vi "MotorDirectControl.vi"(0 "station index":u8, 1 "Hall Positions":i32[](array[numeric]), 3 "JKI_Prefix":string="CMD-", 4 "Exit Refnum":refnum<vi>, 5 "Motion":T3, 6 "PatrType":string, 7 "AnalogData in":dbl[][](array[numeric]), 8 "Manual operation":bool, 9 "open Switch":T1={"Tag Name"="S060.PXI.Signals.PlltData.SN", "Network Path"="172.15.51.1,1,0", "use opc"=FALSE, "DataSocket Reference"={"CWDSLib._DCWDataSocket"=refnum, "CWDSLib._DCWData"=refnum, "OnDataUpdated"=0, "OnStatusUpdated"=0}} {"DataSocket Reference"."OnStatusUpdated" format="%.0x"; "DataSocket Reference"."OnDataUpdated" format="%.0x"}, 10 "test mode":bool, 11 "close Switch":T1={"Tag Name"="S060.PXI.Signals.PlltData.SN", "Network Path"="172.15.51.1,1,0", "use opc"=FALSE, "DataSocket Reference"={"CWDSLib._DCWDataSocket"=refnum, "CWDSLib._DCWData"=refnum, "OnDataUpdated"=0, "OnStatusUpdated"=0}} {"DataSocket Reference"."OnStatusUpdated" format="%.0x"; "DataSocket Reference"."OnDataUpdated" format="%.0x"}, 12 "Position Refnum":refnum<vi>) -> (13 "AnalogData out":dbl[][](array[numeric]), 14 "结果":bool, 15 "Error":string, 18 "motion str":string)   [LabVIEW 2018]
uses:
  02.Type Def's/All Motions.ctl
  05.UserVI's/type defs/plc path and tag.ctl
  <vilib>/Platform/dataskt.llb/DataSocket Reference Type.ctl
  <vilib>/Utility/error.llb/DialogType.ctl
  type def/Direct Value Mode.ctl
panel:
  out "字符串":string
  in  "Display":bool
  in  "参数设定":bool
  out "霍尔位置":i32
  out "波形图表":cluster{"玻璃当前Hall":i64, "玻璃当前Hall":sgl}(graph)
  in  "玻璃一键打开":bool
  in  "玻璃一键关闭":bool
  in  "玻璃点动打开":bool
  in  "玻璃点动关闭":bool
  in  "玻璃初始化":bool
  in  "OK":bool
  in  "打开到位置":bool
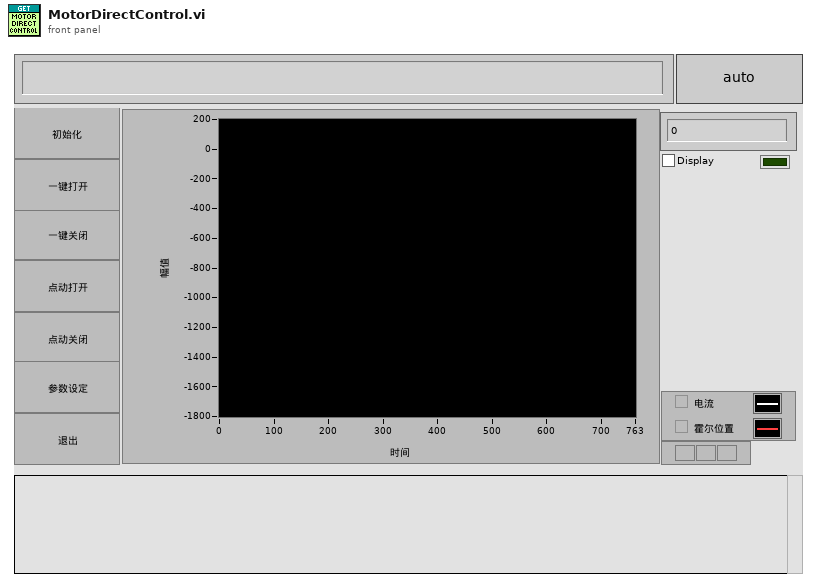
[diagram p1: front panel]
types:
  T1 = typedef "plc path and tag.ctl" = cluster{"Tag Name":string, "Network Path":string, "use opc":bool, "DataSocket Reference":T2}
  T2 = typedef "DataSocket Reference Type.ctl" = cluster{"CWDSLib._DCWDataSocket":refnum<k7>, "CWDSLib._DCWData":refnum<k7>, "OnDataUpdated":u32, "OnStatusUpdated":u32}
  T3 = typedef "All Motions.ctl" = enum16{"Glass Teach", "Glass Slide Open", "Glass Slide Close", "Glass Vent Open", "Glass Vent Close", "Sunshade Teach", "Sunshade Open", "Sunshade Close", "Idle", "Sunshade Open 2", "Sunshade Close 2", "Glass Slide Open Sunshade Open", "Glass Slide Open Sunshade Close", "Glass Slide Close Sunshade Open", "Glass Slide Close Sunshade Close", "Glass Vent Open Sunshade Open", "Glass Vent Open Sunshade Close", "Glass Vent Close Sunshade Open", "Glass Vent Close Sunshade Close", "Express Glass Slide Open", "Express Glass Slide Close", "Express Glass Vent Open", "Express Glass Vent Close", "Express Sunshade Open", "Express Sunshade Close", "Express Sunshade Open 2", "Express Sunshade Close 2", "Express Glass Slide Open Sunshade Open", "Express Glass Slide Open Sunshade Close", "Express Glass Slide Close Sunshade Open", "Express Glass Slide Close Sunshade Close", "Express Glass Vent Open Sunshade Open", "Express Glass Vent Open Sunshade Close", "Express Glass Vent Close Sunshade Open", "Express Glass Vent Close Sunshade Close", "Goto Position Glass", "Goto Position Sunshade", "Sunshade Teach 2"}
  T4 = enum32{"Invalid", "Standard", "Closed", "Hidden", "Minimized", "Maximized"}
  T5 = enum32{"invalid app kind", "Development System", "Run Time System", "Student Edition", "Embedded LabVIEW", "Evaluation", "Custom"}
  T6 = typedef "Direct Value Mode.ctl" = enum16{"Init", "read", "write send cmd", "write ER", "write position", "write AP", "write remote", "write RS", "write all input", "write Msend cmd", "write recevie cmd", "write test mode"}
  T7 = cluster{"Core":cluster{"Current VI Reference":refnum<vi>, "Close Panel on Exit?":bool}, "JKI_Prefix":string, "Hall Positions":i32[], "Action Ref":refnum<user-event>, "DerStationIndex":i32, "RunTime":i32, "Exit Refnum":refnum<vi>, "test state":bool, "current step":string, "Error":string, "Mode":bool, "Manual Operator":bool, "motion string":string, "AnalogData":dbl[][], "station index":i32, "dataNO.":i32, "Position Refnum":refnum<vi>, "Action Switch":T1, "Stop Switch":T1}
  T8 = typedef "DialogType.ctl" = u16
  T9 = cluster{"Current VI Reference":refnum<vi>, "Close Panel on Exit?":bool}
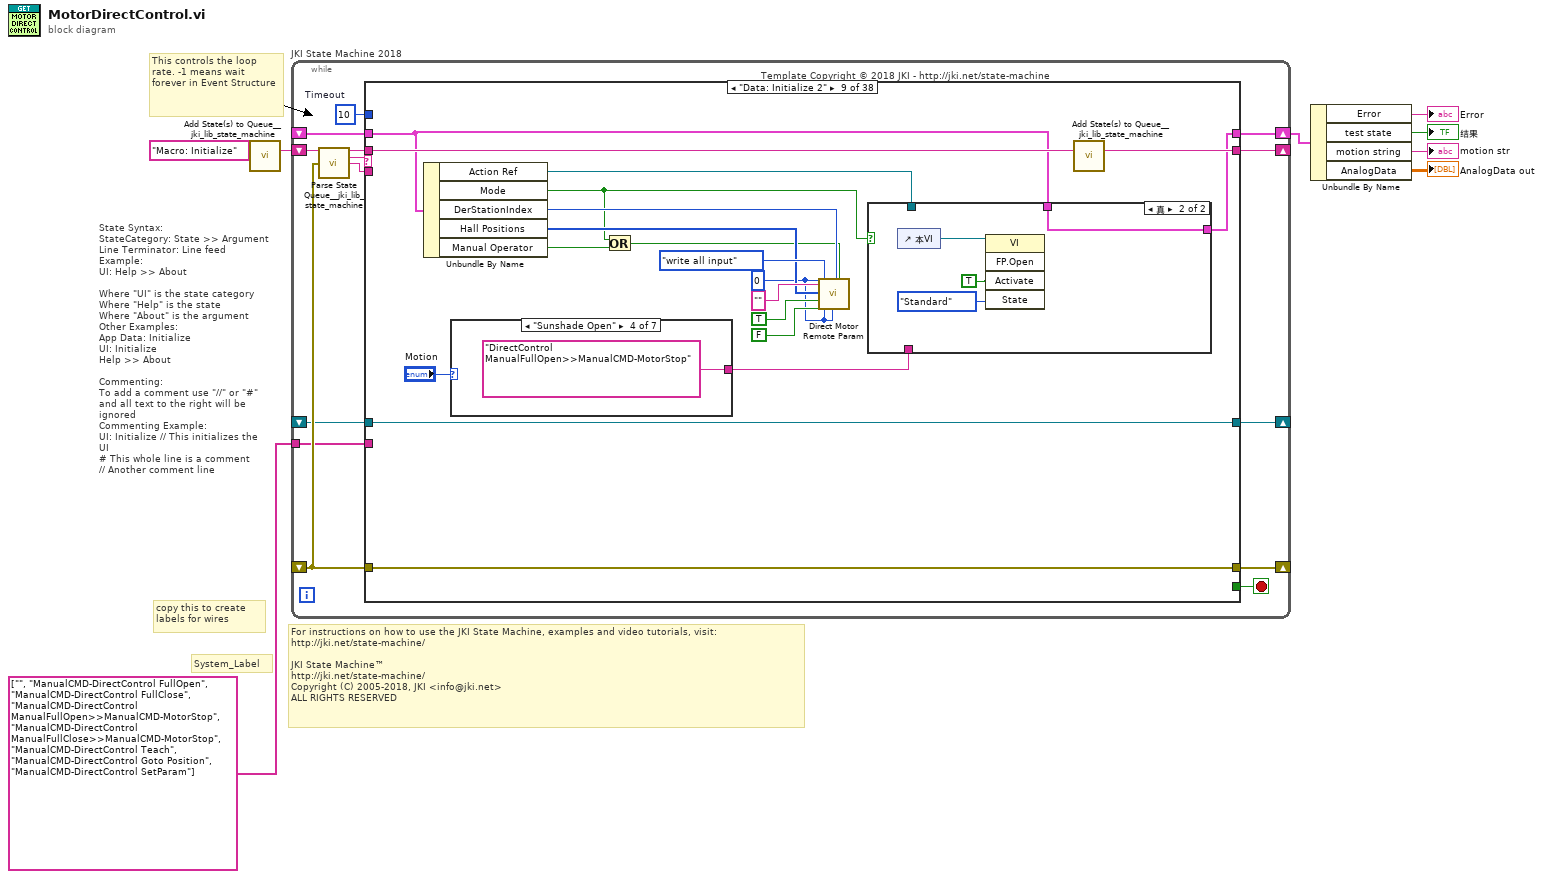
[diagram p0: block diagram]
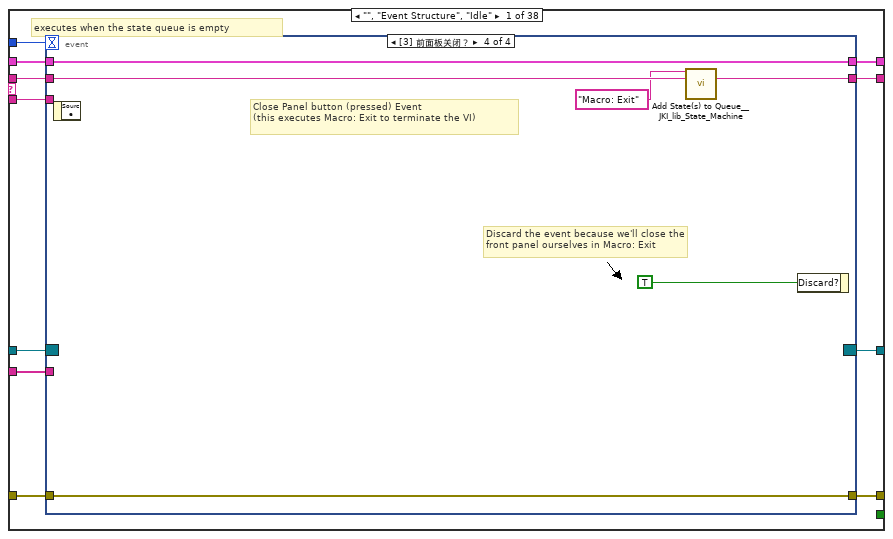
[diagram p2: hidden frame]
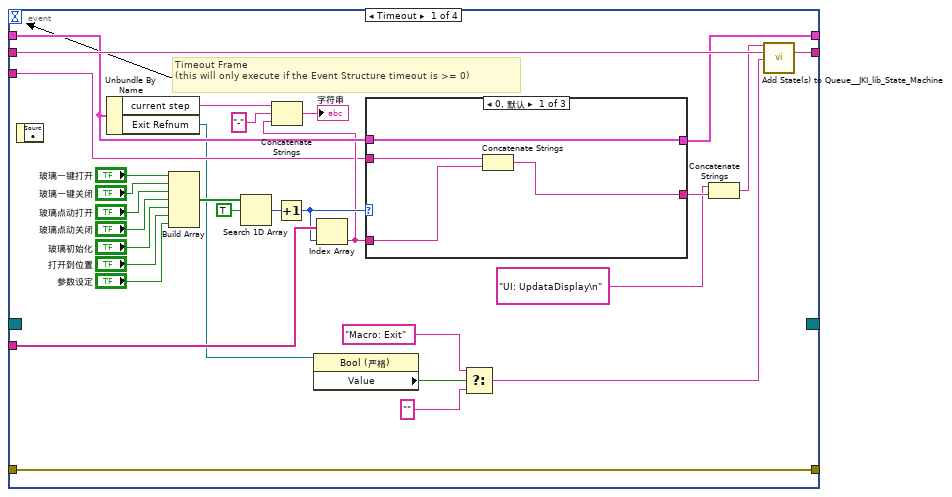
[diagram p3: hidden frame]
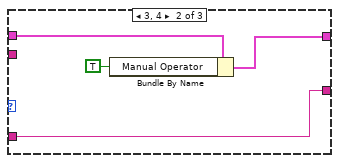
[diagram p4: hidden frame]
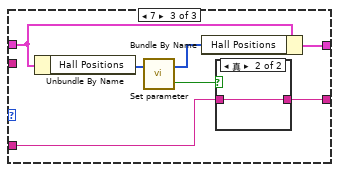
[diagram p5: hidden frame]
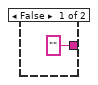
[diagram p6: hidden frame]
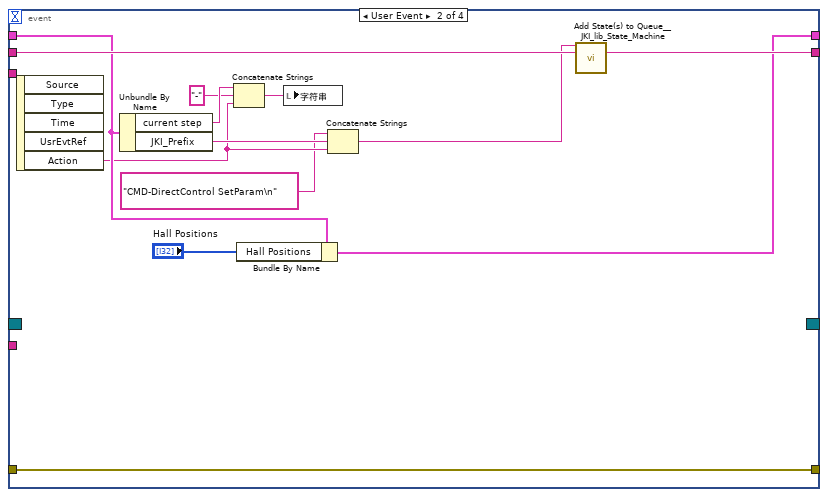
[diagram p7: hidden frame]
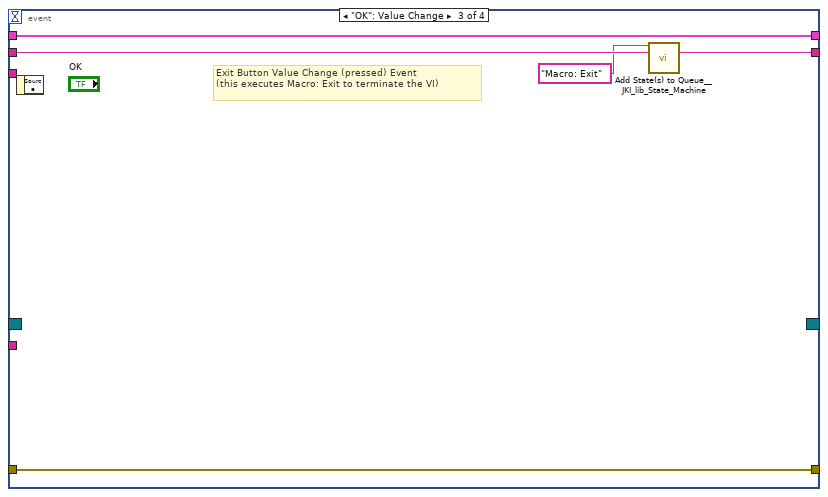
[diagram p8: hidden frame]
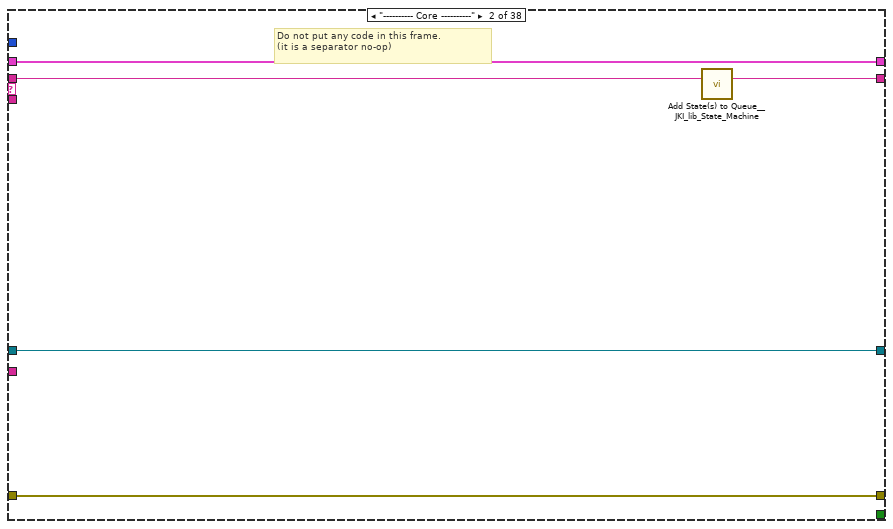
[diagram p9: hidden frame]
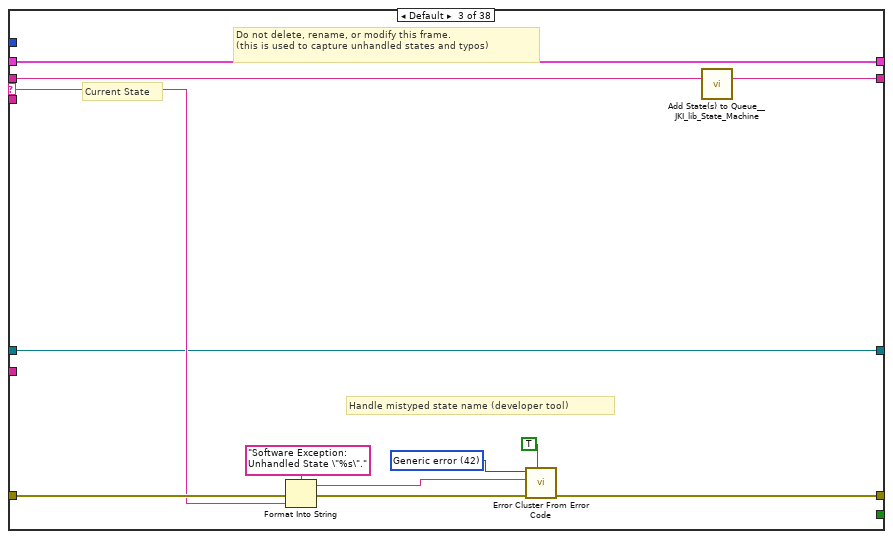
[diagram p10: hidden frame]
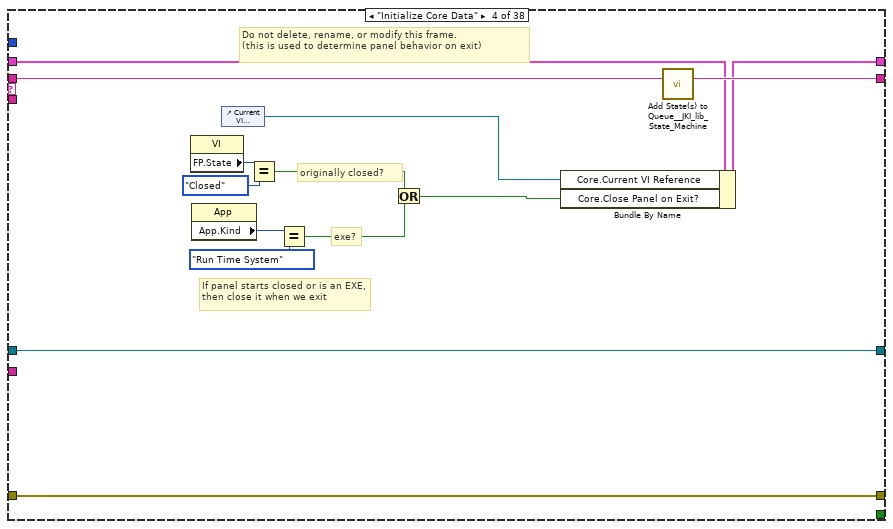
[diagram p11: hidden frame]
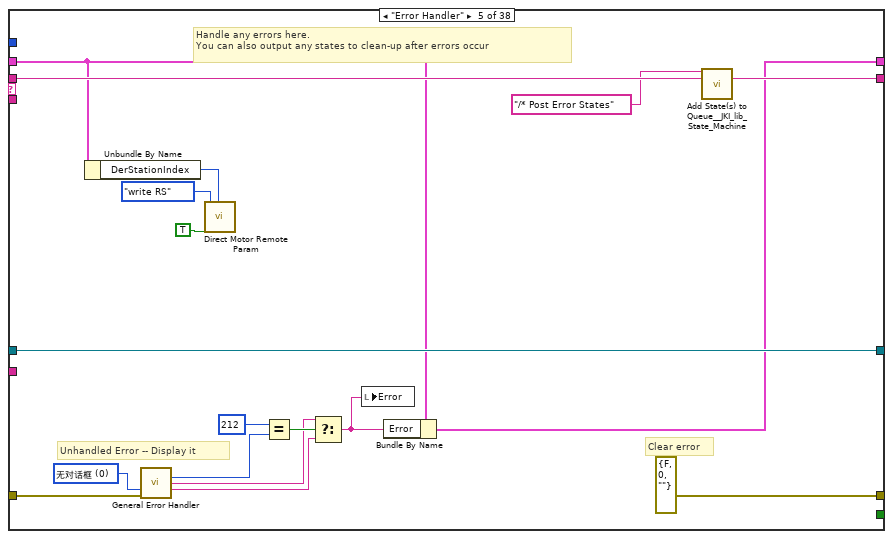
[diagram p12: hidden frame]
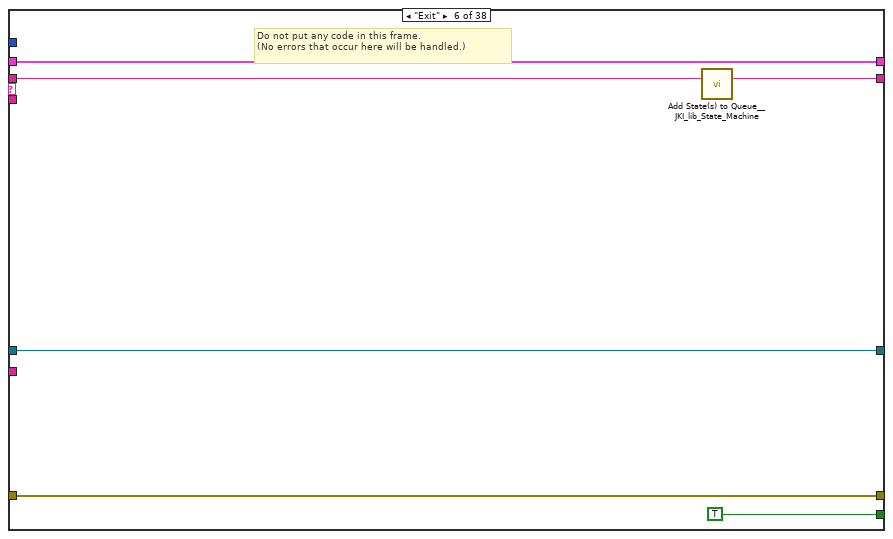
[diagram p13: hidden frame]
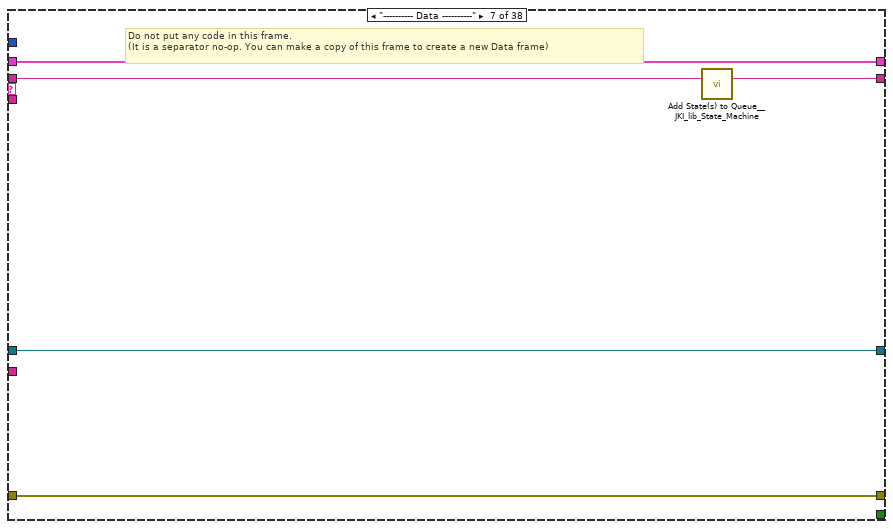
[diagram p14: hidden frame]
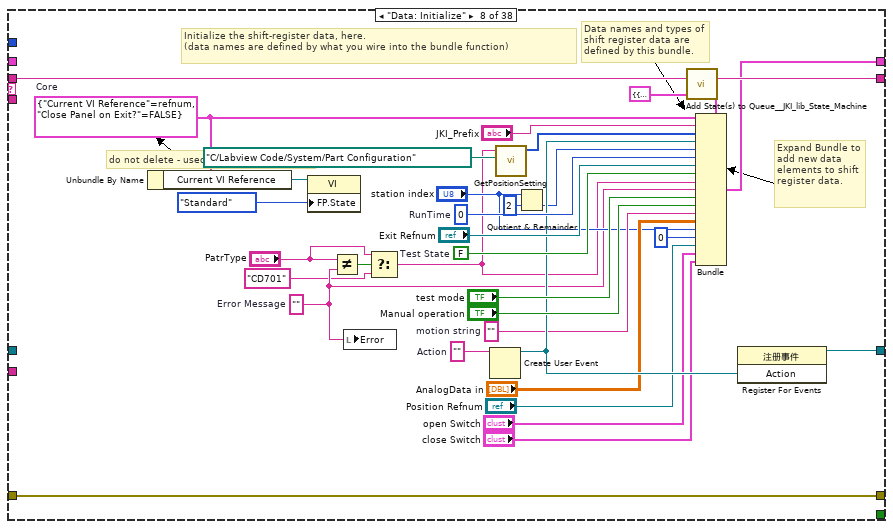
[diagram p15: hidden frame]
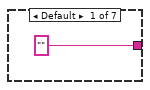
[diagram p16: hidden frame]
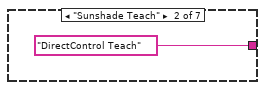
[diagram p17: hidden frame]
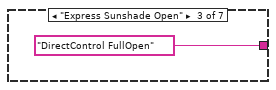
[diagram p18: hidden frame]
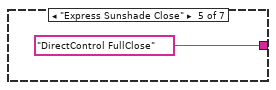
[diagram p19: hidden frame]
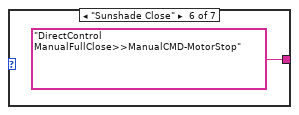
[diagram p20: hidden frame]
diagram:
  # "For instructions on how to use the JKI State Machine, examples and video tutorials, visit:\nhttp://jki.net/state-machine/\n\nJKI State Machine™\nhttp://jki.net/state-machine/\nCopyright (C) 2005-2018, JKI <info@jki.net>\nALL RIGHTS RESERVED"
  # "State Syntax:\nStateCategory: State >> Argument\nLine Terminator: Line feed\nExample:\nUI: Help >> About\n\nWhere \"UI\" is the state category\nWhere \"Help\" is the state\nWhere \"About\" is the argument\nOther Examples:\nApp Data: Initialize\nUI: Initialize\nHelp >> About\n\nCommenting:\nTo add a comment use \"//\" or \"#\" and all text to the right will be ignored\nCommenting Example:\nUI: Initialize // This initializes the UI\n# This whole line is a comment\n// Another comment line"
  # "copy this to create labels for wires"
  # "This controls the loop rate. -1 means wait forever in Event Structure"
  # "System_Label"
  n1 = call <vilib>:"Add State(s) to Queue__jki_lib_state_machine.vi"("State(s) in (\"\")"="Macro: Initialize") -> ("States Out"=w8:string)  [unwired: 14 in]
  n2 = while "JKI State Machine 2018" {
    shift-right: [w15] -> w5
    shift-left: _ -> [w14]
    shift-right: [w18] -> _
    shift-left: _ -> [w12]
    shift-right: [w17] -> _
    shift-left: w8 -> [w19]
    shift-right: [w11] -> _
    shift-left: _ -> [w10]
    tunnel: string[] ["", "ManualCMD-DirectControl FullOpen", "ManualCMD-DirectControl FullClose", "ManualCMD-DirectControl ManualFullOpen>>ManualCMD-MotorStop", "ManualCMD-DirectControl ManualFullClose>>ManualCMD-MotorStop", "ManualCMD-DirectControl Teach", "ManualCMD-DirectControl Goto Position", "ManualCMD-DirectControl SetParam"] -> [w9]
    stop <- w16 stop-if-true
    w13 = 10  # Timeout
    # "Template Copyright © 2018 JKI - http://jki.net/state-machine"
    n3 = call <vilib>:"Parse State Queue__jki_lib_state_machine.vi"("State Queue"=w19, "Error In (no error)"=w12) -> ("Remaining States"=w21:string, "Current State"=w22:string, "Arguments"=w20:string)  [unwired: 11 in]
    n4 = case shown="\"Data: Initialize 2\"" w22 {
      selector: w22 -> [_ _ w111 _ _ _ _ _ _ _ _ _ _ _ _ _ _ _ _ _ _ _ w479 w502 _ _ _ _ _ _ _ _ _ _ _ _ _ _]
      tunnel: w21 -> [w33 w109 w115 w135 w153 w159 w164 w197 w208 w251 w270 w284 w290 w297 w310 w396 w430 w436 w449 w454 w466 w478 w494 w517 w536 w548 w564 w592 w653 w658 w671 w683 w695 w707 w719 w731 w747 w776]
      tunnel: w20 -> [w23 _ _ _ _ _ _ _ _ w238 _ _ _ w292 w304 _ _ _ w438 _ _ _ w485 w507 _ _ _ w570 _ _ _ _ _ _ _ _ _ w749]
      tunnel: w14 -> [w31 w106 w113 w128 w139 w154 w161 _ w207 w247 w272 w281 w288 w295 w306 w390 w427 w434 w446 w451 w458 w470 w488 w511 w528 w544 w560 w585 w656 w659 w668 w674 w686 w698 w710 w727 w743 w769]
      tunnel: [w30 w107 w117 w132 errorcluster {"status"=FALSE, "code"=0, "source"=""} ("error out") w157 w162 w194 w215 w248 w273 w282 w287 w293 w307 w398 w428 errorcluster {"status"=FALSE, "code"=0, "source"=""} ("error out") w447 w452 w464 w476 w492 w515 w534 w546 w562 w577 w654 w660 w669 w681 w693 w705 w717 w729 w745 w761] -> w18
      tunnel: w12 -> [w29 w107 w116 w132 w148 w157 w162 w194 w215 w245 w273 w282 w287 w294 w308 w398 w428 _ w447 w452 w464 w476 w492 w515 w534 w546 w562 w579 w655 w660 w669 w681 w693 w705 w717 w729 w745 w763]
      tunnel: [w32 w108 w114 w134 w152 w158 w163 w196 w209 w250 w271 w283 w289 w296 w309 w397 w429 w435 w448 w453 w465 w477 w493 w516 w535 w547 w563 w591 w652 w661 w670 w682 w694 w706 w718 w730 w746 w775] -> w17
      tunnel: [_ _ _ _ _ TRUE _ _ _ _ _ _ _ _ _ _ _ _ _ _ _ _ _ _ _ _ _ _ _ _ _ _ _ _ _ _ _ _] -> w16
      tunnel: [w28 w106 w113 w133 w141 w154 w161 w195 w206 w247 w272 w281 w288 w295 w306 w389 w427 w434 w446 w451 w456 w469 w486 w509 w526 w542 w558 w584 w656 w659 w668 w672 w684 w697 w708 w725 w741 w768] -> w15
      tunnel: w13 -> [w27 _ _ _ _ _ _ _ _ _ _ _ _ _ _ _ _ _ _ _ _ _ _ _ _ _ _ _ _ _ _ _ _ _ _ _ _ _]
      tunnel: [w25 w105 w110 w122 w149 w155 w160 w193 w216 _ w269 w280 w286 w291 w303 w383 w426 w432 w440 w450 w463 w475 w491 w514 w533 w545 w561 w590 w650 w657 w667 w680 w692 w704 w716 w728 w744 w774] -> w11
      tunnel: w10 -> [w26 w105 w110 w122 w149 w155 w160 _ w216 w246 w269 w280 w286 w291 w303 w383 w426 w432 w440 w450 w463 w475 w491 w514 w533 w545 w561 w590 w650 w657 w667 w680 w692 w704 w716 w728 w744 w774]
      tunnel: w9 -> [w24 _ _ _ _ _ _ _ _ _ _ _ _ _ _ _ _ _ _ _ _ _ _ _ _ _ _ _ _ _ _ _ _ _ _ _ _ _]
      frame "", "Event Structure", "Idle" {
        # "executes when the state queue is empty"
        n5 = event shown="[3] 前面板关闭？" {
          selector: w26 -> [_ _ _ _]
          dyn-events: [_ _ _ _] -> w25
          timeout: w27 -> [_ _ _ _]
          tunnel: w33 -> [w63 w92 w98 w104]
          tunnel: [w62 w91 w97 w103] -> w32
          tunnel: w31 -> [w44 w89 w95 w101]
          tunnel: [w61 w93 w96 w102] -> w30
          tunnel: w29 -> [w61 w93 w96 w102]
          tunnel: [w48 w88 w95 w101] -> w28
          tunnel: w24 -> [w50 _ _ _]
          tunnel: w23 -> [w39 _ _ _]
          event Timeout {
            # "Timeout Frame\n(this will only execute if the Event Structure timeout is >= 0)"
            n6 = event-data() -> ()  [unwired: 1 in, 1 out]
            n7 = Unbundle By Name(w44) -> ("current step"=w43:string, "Exit Refnum"=w38:refnum<vi>)
            n8 = Build Array("玻璃一键打开", "玻璃一键关闭", "玻璃点动打开", "玻璃点动关闭", "玻璃初始化", "打开到位置", "参数设定") -> (w59:bool[])
            n9 = Search 1D Array(1D array=w59, element=TRUE ("元素")) -> (index of element=w54:i32)  [unwired: 1 in]
            n10 = Increment(x=w54) -> (x+1=w49:i32)
            n11 = property class="Bool (严格)"(reference=w38) -> ("Value"=w37:bool)  [unwired: 1 in, 2 out]
            n12 = Index Array(array=w50, index=w49) -> (element=w41:string)
            n13 = Concatenate Strings(w43, "-", w41) -> (→"字符串":string)
            n14 = case shown="0, 默认" w49 {
              tunnel: w41 -> [w65 w71 w78]
              tunnel: [w64 w71 w77] -> w47
              tunnel: w44 -> [w67 w70 w75]
              tunnel: [w67 w68 w72] -> w48
              tunnel: w39 -> [w66 _ _]
              frame 0, Default {
                n15 = Concatenate Strings(w66, w65) -> (w64:string)
              }
              frame 3, 4 {
                n16 = Bundle By Name(cluster=w70, "Manual Operator"=TRUE) -> (w68:T7)
              }
              frame 7 {
                n17 = Unbundle By Name(w75) -> ("Hall Positions"=w74:i32[])
                n18 = call "Set parameter.vi"("霍尔参数"=w74) -> ("设定"=w76:bool, "输出参数"=w73:u16[])  [unwired: 1 in]
                n19 = Bundle By Name(cluster=w75, "Hall Positions"=w73) -> (w72:T7)
                n20 = case shown="真" w76 {
                  tunnel: w78 -> [_ w80]
                  tunnel: ["" w80] -> w77
                  frame False {
                  }
                  frame True {
                  }
                }
              }
            }
            n21 = Select(t="Macro: Exit", s=w37, f="") -> (s? t:f=w34:string)
            n22 = Concatenate Strings("UI: UpdataDisplay\n", w47) -> (w45:string)
            n23 = call <vilib>:"Add State(s) to Queue__JKI_lib_State_Machine.vi"("State(s) in Front (\"\")"=w45, "State(s) in (\"\")"=w63, "State(s) at Back (\"\")"=w34) -> ("States Out"=w62:string)  [unwired: 12 in]
          }
          event User Event {
            n24 = event-data() -> ("Action"=w85:string)  [unwired: 1 in, 4 out]
            n25 = Unbundle By Name(w89) -> ("current step"=w86:string, "JKI_Prefix"=w90:string)
            n26 = Concatenate Strings(w86, "-", w85) -> (w83:string)
            n27 = Bundle By Name(cluster=w89, "Hall Positions"="Hall Positions") -> (w88:T7)
            n28 = local write "字符串"(w83) -> ()
            n29 = Concatenate Strings("CMD-DirectControl SetParam\n", w90, w85) -> (w87:string)
            n30 = call <vilib>:"Add State(s) to Queue__JKI_lib_State_Machine.vi"("State(s) in Front (\"\")"=w87, "State(s) in (\"\")"=w92) -> ("States Out"=w91:string)  [unwired: 13 in]
          }
          event "OK": Value Change {
            # "Exit Button Value Change (pressed) Event\n(this executes Macro: Exit to terminate the VI)"
            n31 = event-data() -> ()  [unwired: 1 in, 1 out]
            n32 = call <vilib>:"Add State(s) to Queue__JKI_lib_State_Machine.vi"("State(s) in Front (\"\")"="Macro: Exit", "State(s) in (\"\")"=w98) -> ("States Out"=w97:string)  [unwired: 13 in]
          }
          event Panel Close? {
            # "Discard the event because we'll close the front panel ourselves in Macro: Exit"
            # "Close Panel button (pressed) Event\n(this executes Macro: Exit to terminate the VI)"
            n33 = event-data() -> ()  [unwired: 1 in, 1 out]
            n34 = call <vilib>:"Add State(s) to Queue__JKI_lib_State_Machine.vi"("State(s) in Front (\"\")"="Macro: Exit", "State(s) in (\"\")"=w104) -> ("States Out"=w103:string)  [unwired: 13 in]
            n35 = event-data("Discard?"=TRUE) -> ()  [unwired: 1 in, 1 out]
          }
        }
      }
      frame "---------- Core ----------" {
        # "Do not put any code in this frame.\n(it is a separator no-op)"
        n36 = call <vilib>:"Add State(s) to Queue__JKI_lib_State_Machine.vi"("State(s) in (\"\")"=w109) -> ("States Out"=w108:string)  [unwired: 14 in]
      }
      frame Default {
        w120 = 42 items=["No error", "Argument error", "Memory is full", "Out of zone", "End of file", "File already open", "Generic file I/O error", "File not found", "File permission error", "Disk is full", "Duplicate path", "Too many files open", "System feature not enabled", "Resource file not found", "Cannot add resource", "Resource not found", "Image not found", "Image memory error", "Pen does not exist", "Config type invalid", "Config token not found", "Config parse error", "Config memory error", "Bad external code format", "Bad external code offset", "External code not present", "Null window", "Destroy window error", "Null menu", "Print aborted", "Bad print record", "Print driver error", "Windows error during printing", "Memory error during printing", "Print dialog error", "Generic print error", "Invalid device refnum", "Device not found", "Device parameter error", "Device unit error", "Cannot open device", "Device call aborted", "Generic error", "Cancelled by user", "Object ID too low", "Object ID too high", "Object not in heap", "Unknown heap", "Unknown object (invalid DefProc)", "Unknown object (DefProc not in table)", "Message out of range", "Invalid (null) method", "Unknown message", "Manager call not supported", "Bad address", "Network operation in progress", "Network operation timed out", "Connection is busy", "Network attribute not supported", "Network error", "Address in use", "System out of memory", "Connection aborted", "Connection refused", "Not connected", "Already connected", "Connection closed", "Initialization error (interapplication manager)", "Bad occurrence", "Wait on unbound occurrence handler", "Occurrence queue overflow", "Datalog type conflict", "Unused", "Unrecognized type (interapplication manager)", "Memory corrupt", "Failed to make temporary DLL", "Old CIN version", "Drag socket not found", "Failed to load drop-object", "Failed to register OLE object", "Failed to release OLE object", "Format specifier type mismatch", "Unknown format specifier", "Too few format specifiers", "Too many format specifiers", "Scan failed", "Newer CIN version", "Error converting to variant", "Runtime menu error", "Password tampered", "Variant attribute not found", "Incompatible variant data type", "Event data is not available", "Event Store is not present", "Occurrence is not found", "Event Queue is not created", "Event info is not available", "Refnum passed is NULL", "Error retrieving Class GUID", "Error retrieving CoClass GUID", "Error retrieving TypeLib GUID.", "Bad built application magic bytes.", "Specific driver is different from the specific driver associated with the Logical Name.", "There is no session opened to the class driver.", "Max Error", "MAX - Error with config objects", "MAX - Error loading configuration", "MAX - Group not supported"]
        # "Current State"
        # "Do not delete, rename, or modify this frame.\n(this is used to capture unhandled states and typos)"
        # "Handle mistyped state name (developer tool)"
        n37 = Format Into String(format string="Software Exception: Unhandled State \"%s\"." ("message"), error in=w116, w111) -> (resulting string=w119:string, error out=w118:errorcluster)  [unwired: 1 in]
        n38 = call <vilib>:"Error Cluster From Error Code.vi"("show call chain? (False)"=TRUE, "error in (no error)"=w118, "error message (\"\")"=w119, "error code (0)"=w120) -> ("error out"=w117:errorcluster)  [unwired: 5 in]
        n39 = call <vilib>:"Add State(s) to Queue__JKI_lib_State_Machine.vi"("State(s) in (\"\")"=w115) -> ("States Out"=w114:string)  [unwired: 14 in]
      }
      frame "Initialize Core Data" {
        # "Do not delete, rename, or modify this frame.\n(this is used to determine panel behavior on exit)"
        # "originally closed?"
        # "exe?"
        # "If panel starts closed or is an EXE, then close it when we exit"
        n40 = property class="VI"() -> ("FP.State"=w125:T4)  [unwired: 2 in, 2 out]
        n41 = property class="App"() -> ("App.Kind"=w131:T5)  [unwired: 2 in, 2 out]
        n42 = control-ref of="Current VI Reference"() -> (w126:refnum<vi>)
        n43 = Equal?(x=w125, y=T4."Closed" ("Front Panel Window:State")) -> (x = y?=w123:bool)
        n44 = Equal?(x=w131, y=T5."Run Time System" ("Application:Kind")) -> (x = y?=w129:bool)
        n45 = Or(x=w123, y=w129) -> (x .or. y?=w127:bool)
        n46 = Bundle By Name(cluster=w128, "Core.Current VI Reference"=w126, "Core.Close Panel on Exit?"=w127) -> (w133:T7)
        n47 = call <vilib>:"Add State(s) to Queue__JKI_lib_State_Machine.vi"("State(s) in (\"\")"=w135) -> ("States Out"=w134:string)  [unwired: 14 in]
      }
      frame "Error Handler" {
        w142 = T8 0 items=["无对话框", "确定信息", "继续或停止信息", "确定信息＋警告", "继续/停止+警告"] ("type of dialog (OK msg:1)")
        # "Unhandled Error -- Display it"
        # "Handle any errors here.\nYou can also output any states to clean-up after errors occur"
        # "Clear error"
        n48 = Unbundle By Name(w139) -> ("DerStationIndex"=w138:i32)
        n49 = call <vilib>:"General Error Handler.vi"("type of dialog (OK msg:1)"=w142, "error in (no error)"=w148) -> ("code out"=w147:i32, "source out"=w144:string, "message"=w143:string)  [unwired: 9 in, 2 out]
        n50 = call "Direct Motor Remote Param.vi"("remote Stop in"=TRUE, "mode"=Direct_Value_Mode."write RS", "工位数"=w138) -> ()  [unwired: 16 in, 9 out]
        n51 = Equal?(x=212, y=w147) -> (x = y?=w145:bool)
        n52 = Select(t=w144, s=w145, f=w143) -> (s? t:f=w140:string)
        n53 = local write "Error"(w140) -> ()
        n54 = Bundle By Name(cluster=w139, "Error"=w140) -> (w141:T7)
        n55 = call <vilib>:"Add State(s) to Queue__JKI_lib_State_Machine.vi"("State(s) in Front (\"\")"="/* Post Error States", "State(s) in (\"\")"=w153) -> ("States Out"=w152:string)  [unwired: 13 in]
      }
      frame "Exit" {
        # "Do not put any code in this frame.\n(No errors that occur here will be handled.)"
        n56 = call <vilib>:"Add State(s) to Queue__JKI_lib_State_Machine.vi"("State(s) in (\"\")"=w159) -> ("States Out"=w158:string)  [unwired: 14 in]
      }
      frame "---------- Data ----------" {
        # "Do not put any code in this frame.\n(It is a separator no-op. You can make a copy of this frame to create a new Data frame)"
        n57 = call <vilib>:"Add State(s) to Queue__JKI_lib_State_Machine.vi"("State(s) in (\"\")"=w164) -> ("States Out"=w163:string)  [unwired: 14 in]
      }
      frame "Data: Initialize" {
        w181 = ""  # motion string
        w185 = ""  # Action
        w166 = ""  # Error Message
        w188 = FALSE  # Test State
        w190 = 0  # RunTime
        w175 = T9 {"Current VI Reference"=refnum, "Close Panel on Exit?"=FALSE}  # Core
        # "do not delete - used by framework"
        # "Expand Bundle to add new data elements to shift register data."
        # "Data names and types of shift register data are defined by this bundle."
        # "Initialize the shift-register data, here.\n(data names are defined by what you wire into the bundle function)"
        n58 = Unbundle By Name(w175) -> ("Current VI Reference"=w174:refnum<vi>)
        n59 = property class="VI"(reference=w174, "FP.State"=T4."Standard" ("前面板窗口:状态")) -> ()  [unwired: 1 in, 2 out]
        n60 = Not Equal?(x="PatrType", y=w166) -> (x != y?=w169:bool)
        n61 = local write "Error"(w166) -> ()
        n62 = Select(t="PatrType", s=w169, f="CD701") -> (s? t:f=w167:string)
        n63 = Create User Event(user event datatype=w185) -> (user event=w184:refnum<user-event>)  [unwired: 1 in, 1 out]
        n64 = call "GetPositionSetting.vi"("基路径"=path "C:/Labview Code/System/Part Configuration", "Part Type"=w167) -> ("Hall Positions"=w171:i32[])  [unwired: 9 in]
        n65 = Quotient & Remainder(x="station index", y=u8 2) -> (floor(x/y)=w182:u8)  [unwired: 1 out]
        n66 = call <vilib>:"Add State(s) to Queue__JKI_lib_State_Machine.vi"("State(s) in (\"\")"=w197) -> ("States Out"=w196:string)  [unwired: 14 in]
        n67 = Bundle(cluster=T7 {"Core"={"Current VI Reference"=refnum, "Close Panel on Exit?"=FALSE}, "JKI_Prefix"="", "Hall Positions"=[], "Action Ref"=refnum, "DerStationIndex"=0, "RunTime"=0, "Exit Refnum"=refnum, "test state"=FALSE, "current step"="", "Error"="", "Mode"=FALSE, "Manual Operator"=FALSE, "motion string"="", "AnalogData"=[], "station index"=0, "dataNO."=0, "Position Refnum"=refnum, "Action Switch"={"Tag Name"="CD701.ST3.ST45_EOL Sunshade Open Switch", "Network Path"="opc://localhost/National Instruments.NIOPCServers.V5/", "use opc"=TRUE, "DataSocket Reference"={"CWDSLib._DCWDataSocket"=refnum, "CWDSLib._DCWData"=refnum, "OnDataUpdated"=2941255746, "OnStatusUpdated"=2940207171}}, "Stop Switch"={"Tag Name"="CD701.ST3.ST45_EOL Sunshade Open Switch", "Network Path"="opc://localhost/National Instruments.NIOPCServers.V5/", "use opc"=TRUE, "DataSocket Reference"={"CWDSLib._DCWDataSocket"=refnum, "CWDSLib._DCWData"=refnum, "OnDataUpdated"=2941255746, "OnStatusUpdated"=2940207171}}} ("簇"), "Core"=w175, "JKI_Prefix"="JKI_Prefix", "Hall Positions"=w171, "Action Ref"=w184, "DerStationIndex"=w182, "RunTime"=w190, "Exit Refnum"="Exit Refnum", "test state"=w188, "current step"=w167, "Error"=w166, "Mode"="test mode", "Manual Operator"="Manual operation", "motion string"=w181, "AnalogData"="AnalogData in", "station index"="station index", "dataNO."=0, "Position Refnum"="Position Refnum", "Action Switch"="open Switch", "Stop Switch"="close Switch") -> (w195:T7)
        n68 = register-events(w184) -> (reference out=w193:refnum<event-registration>)  [unwired: 2 in, 1 out]
      }
      frame "Data: Initialize 2" {
        w202 = u32 0 ("cmd in")
        n69 = Unbundle By Name(w207) -> ("Action Ref"=w201:refnum<user-event>, "Mode"=w199:bool, "DerStationIndex"=w214:i32, "Hall Positions"=w203:i32[], "Manual Operator"=w200:bool)
        n70 = case shown="\"Sunshade Open\"" "Motion" {
          tunnel: ["" "DirectControl Teach" "DirectControl FullOpen" "DirectControl ManualFullOpen>>ManualCMD-MotorStop" "DirectControl FullClose" "DirectControl ManualFullClose>>ManualCMD-MotorStop" "DirectControl Goto Position"] -> w205
          frame Default {
          }
          frame "Sunshade Teach" {
          }
          frame "Express Sunshade Open" {
          }
          frame "Sunshade Open" {
          }
          frame "Express Sunshade Close" {
          }
          frame "Sunshade Close" {
          }
          frame "Goto Position Sunshade" {
          }
        }
        n71 = Or(x=w199, y=w200) -> (x .or. y?=w198:bool)
        n72 = call "Direct Motor Remote Param.vi"("send cmd in"=w202, "ErrorString in"="", "position in"=w203, "remote in"=TRUE, "remote Stop in"=FALSE, "mode"=Direct_Value_Mode."write all input", "M-send cmd in"=w202, "recevie cmd in"=w202, "index"=w214, "test mode in(T:manual)"=w198) -> ()  [unwired: 9 in, 9 out]
        n73 = case shown="真" w199 {
          tunnel: w201 -> [w228 _]
          tunnel: w207 -> [w227 w232]
          tunnel: [w225 w232] -> w206
          tunnel: w205 -> [w224 _]
          frame False {
            n74 = Generate User Event(user event=w228, event data cluster=w224) -> (user event out=w226:refnum<user-event>)  [unwired: 2 in, 1 out]
            n75 = Bundle By Name(cluster=w227, "Action Ref"=w226) -> (w225:T7)
          }
          frame True {
            n76 = control-ref of="本VI"() -> (w229:refnum<vi>)
            n77 = invoke class="VI" method="FP.Open"(reference=w229, "Activate"=TRUE ("激活？"), "State"=T4."Standard" ("状态")) -> ()  [unwired: 2 in, 5 out]
          }
        }
        n78 = call <vilib>:"Add State(s) to Queue__jki_lib_state_machine.vi"("State(s) in (\"\")"=w208) -> ("States Out"=w209:string)  [unwired: 14 in]
      }
      frame "Data: Cleanup" {
        w240 = u32 0 ("cmd in")
        # "Cleanup any data and references, here.\n(this is called automatically, by the Macro: Exit)"
        n79 = Unbundle By Name(w247) -> ("DerStationIndex"=w233:i32, "Core.Current VI Reference"=w249:refnum<vi>, "Manual Operator"=w239:bool, "Position Refnum"=w235:refnum<vi>, "test state"=w234:bool)
        n80 = Unregister For Events(event registration refnum=w246, error in=w245) -> (error out=w244:errorcluster)
        n81 = Close Reference(reference=w249, error in (no error)=w244) -> (error out=w248:errorcluster)
        n82 = case shown="真" w239 {
          tunnel: w233 -> [w264 w268]
          tunnel: w240 -> [w263 w266]
          frame False {
            n83 = call "Direct Motor Remote Param.vi"("send cmd in"=w263, "mode"=Direct_Value_Mode."write send cmd", "index"=w264) -> ()  [unwired: 16 in, 9 out]
          }
          frame True {
            n84 = call "Direct Motor Remote Param.vi"("mode"=Direct_Value_Mode."write Msend cmd", "M-send cmd in"=w266, "index"=w268) -> ()  [unwired: 16 in, 9 out]
          }
        }
        n85 = Equal?(x=w238, y="0x50") -> (x = y?=w236:bool)
        n86 = case shown="真" w236 {
          tunnel: w235 -> [_ w252]
          tunnel: w234 -> [_ w260]
          tunnel: w233 -> [_ w256]
          frame False {
          }
          frame True {
            n87 = Boolean To (0,1)(Boolean=w260) -> (0, 1=w259:i16)
            n88 = call "Direct Motor Remote Param.vi"("mode"=Direct_Value_Mode."read", "index"=w256) -> ("actual pos out"=w254:i64)  [unwired: 17 in, 8 out]
            n89 = Bundle("ST", w259) -> (w258:cluster{string, i16})  [unwired: 1 in]
            n90 = Bundle("Position", "actual pos out"=w254) -> (w253:cluster{string, "actual pos out":i64})  [unwired: 1 in]
            n91 = Build Array(w253, w258) -> (w262:cluster{string, "actual pos out":i64}[])
            n92 = property class="Ctl"(reference=w252, "Value"=w262) -> ()  [unwired: 1 in, 2 out]
          }
        }
        n93 = call "Direct Motor Remote Param.vi"("remote in"=FALSE, "mode"=Direct_Value_Mode."write remote", "index"=w233) -> ()  [unwired: 16 in, 9 out]
        n94 = call <vilib>:"Add State(s) to Queue__JKI_lib_State_Machine.vi"("State(s) in (\"\")"=w251) -> ("States Out"=w250:string)  [unwired: 14 in]
        n95 = call "Direct Motor Remote Param.vi"("mode"=Direct_Value_Mode."write recevie cmd", "工位数"=w233, "recevie cmd in"=w240) -> ()  [unwired: 16 in, 9 out]
      }
      frame "Data: UI-Cleanup" {
        n96 = flat-sequence {
          tunnel: w272 -> [w277]
          frame #0 {
            w274 = u32 0 ("cmd in")
            n97 = Unbundle By Name(w277) -> ("DerStationIndex"=w276:i32)
            n98 = call "Direct Motor Remote Param.vi"("mode"=Direct_Value_Mode."write Msend cmd", "M-send cmd in"=w274, "index"=w276) -> ()  [unwired: 16 in, 9 out]
            n99 = call "Direct Motor Remote Param.vi"("mode"=Direct_Value_Mode."write recevie cmd", "工位数"=w276, "recevie cmd in"=w274) -> ()  [unwired: 16 in, 9 out]
          }
          frame #1 {
            n100 = Wait (ms)(milliseconds to wait=u32 300 ("毫秒计时值")) -> ()  [unwired: 1 out]
          }
        }
        n101 = call <vilib>:"Add State(s) to Queue__JKI_lib_State_Machine.vi"("State(s) in (\"\")"=w270) -> ("States Out"=w271:string)  [unwired: 14 in]
      }
      frame "---------- UI ----------" {
        # "Do not put any code in this frame.\n(It is a separator no-op. You can make a copy of this frame to create a new UI frame)"
        n102 = call <vilib>:"Add State(s) to Queue__JKI_lib_State_Machine.vi"("State(s) in (\"\")"=w284) -> ("States Out"=w283:string)  [unwired: 14 in]
      }
      frame "UI: Initialize" {
        # "Initialize the User Interface, here.\n(this is called automatically, by the Macro: Init)"
        n103 = property on="波形图表" class="WFChart (严格)"("History Data"=cluster{"玻璃当前Hall":i64, "玻璃当前Hall":sgl}[] [] ("历史数据")) -> ()  [unwired: 2 in, 2 out]
        n104 = call <vilib>:"Add State(s) to Queue__JKI_lib_State_Machine.vi"("State(s) in (\"\")"=w290) -> ("States Out"=w289:string)  [unwired: 14 in]
      }
      frame "UI: Cursor Set" {
        # "Argument"
        # "Set and Unset Cursor Busy.\n(Usage: \"UI: Cursor Set >> Busy|Idle\")"
        n105 = case shown="\"Idle\", 默认" w292 {
          tunnel: w294 -> [w299 w301]
          tunnel: [w298 w300] -> w293
          frame "Idle", Default {
            n106 = call <vilib>:"Unset Busy.vi"("error in (no error)"=w299) -> ("error out"=w298:errorcluster)  [unwired: 10 in]
          }
          frame "Busy" {
            n107 = call <vilib>:"Set Busy.vi"("error in (no error)"=w301) -> ("error out"=w300:errorcluster)  [unwired: 9 in, 1 out]
          }
        }
        n108 = call <vilib>:"Add State(s) to Queue__JKI_lib_State_Machine.vi"("State(s) in (\"\")"=w297) -> ("States Out"=w296:string)  [unwired: 14 in]
      }
      frame "UI: Front Panel State" {
        # "Argument"
        # "Set Front Panel Open or Closed\n(Usage: \"UI: Front Panel State >> Open|Close\")"
        n109 = Unbundle By Name(w306) -> ("Core.Current VI Reference"=w305:refnum<vi>, "Mode"=w302:bool)
        n110 = case shown="真" w302 {
          tunnel: w308 -> [w311 w315]
          tunnel: [w311 w314] -> w307
          tunnel: w305 -> [_ w313]
          tunnel: w304 -> [_ w312]
          frame False {
          }
          frame True {
            n111 = case shown="\"Close\", \"Closed\"" w312 {
              tunnel: w315 -> [w321 w336 w347 w360 w373]
              tunnel: [w323 w337 w349 w362 w375] -> w314
              tunnel: w313 -> [w322 w334 w348 w361 w374]
              frame "Open", "Standard", Default {
                w316 = T4."Standard" ("State")
                n112 = property class="VI"(reference=w322, error in=w321) -> (reference out=w319:refnum<vi>, error out=w320:errorcluster, "FP.State"=w318:T4)
                n113 = Not Equal?(x=w318, y=w316) -> (x != y?=w317:bool)
                n114 = case shown="假" w317 {
                  tunnel: [w327 w329] -> w323
                  tunnel: w320 -> [w326 w329]
                  tunnel: w319 -> [w325 _]
                  tunnel: w316 -> [w324 _]
                  frame True {
                    n115 = invoke class="VI" method="FP.Open"(reference=w325, error in=w326, "Activate"=TRUE, "State"=w324) -> (error out=w327:errorcluster)  [unwired: 1 in, 4 out]
                  }
                  frame False {
                  }
                }
              }
              frame "Close", "Closed" {
                n116 = property class="VI"(reference=w334, error in=w336) -> (reference out=w333:refnum<vi>, error out=w335:errorcluster, "FP.State"=w331:T4)
                n117 = Not Equal?(x=w331, y=T4."Closed" ("Front Panel Window:State")) -> (x != y?=w330:bool)
                n118 = case shown="真" w330 {
                  tunnel: [w338 w341] -> w337
                  tunnel: w335 -> [w338 w340]
                  tunnel: w333 -> [_ w339]
                  frame False {
                  }
                  frame True {
                    n119 = invoke class="VI" method="FP.Close"(reference=w339, error in=w340) -> (error out=w341:errorcluster)  [unwired: 1 in, 2 out]
                  }
                }
              }
              frame "Hidden", "Hide" {
                w342 = T4."Hidden" ("State")
                n120 = property class="VI"(reference=w348, error in=w347) -> (reference out=w345:refnum<vi>, error out=w346:errorcluster, "FP.State"=w344:T4)
                n121 = Not Equal?(x=w344, y=w342) -> (x != y?=w343:bool)
                n122 = case shown="真" w343 {
                  tunnel: [w353 w354] -> w349
                  tunnel: w346 -> [w352 w354]
                  tunnel: w345 -> [w351 _]
                  tunnel: w342 -> [w350 _]
                  frame True {
                    n123 = invoke class="VI" method="FP.Open"(reference=w351, error in=w352, "State"=w350) -> (error out=w353:errorcluster)  [unwired: 2 in, 4 out]
                  }
                  frame False {
                  }
                }
              }
              frame "Minimize", "Minimized" {
                w355 = T4."Minimized" ("State")
                n124 = property class="VI"(reference=w361, error in=w360) -> (reference out=w358:refnum<vi>, error out=w359:errorcluster, "FP.State"=w357:T4)
                n125 = Not Equal?(x=w357, y=w355) -> (x != y?=w356:bool)
                n126 = case shown="真" w356 {
                  tunnel: [w366 w367] -> w362
                  tunnel: w359 -> [w365 w367]
                  tunnel: w358 -> [w364 _]
                  tunnel: w355 -> [w363 _]
                  frame True {
                    n127 = invoke class="VI" method="FP.Open"(reference=w364, error in=w365, "State"=w363) -> (error out=w366:errorcluster)  [unwired: 2 in, 4 out]
                  }
                  frame False {
                  }
                }
              }
              frame "Maximize", "Maximized" {
                w368 = T4."Maximized" ("State")
                n128 = property class="VI"(reference=w374, error in=w373) -> (reference out=w371:refnum<vi>, error out=w372:errorcluster, "FP.State"=w370:T4)
                n129 = Not Equal?(x=w370, y=w368) -> (x != y?=w369:bool)
                n130 = case shown="真" w369 {
                  tunnel: [w379 w380] -> w375
                  tunnel: w372 -> [w378 w380]
                  tunnel: w371 -> [w377 _]
                  tunnel: w368 -> [w376 _]
                  frame True {
                    n131 = invoke class="VI" method="FP.Open"(reference=w377, error in=w378, "State"=w376) -> (error out=w379:errorcluster)  [unwired: 2 in, 4 out]
                  }
                  frame False {
                  }
                }
              }
            }
          }
        }
        n132 = call <vilib>:"Add State(s) to Queue__JKI_lib_State_Machine.vi"("State(s) in (\"\")"=w310) -> ("States Out"=w309:string)  [unwired: 14 in]
      }
      frame "UI: UpdataDisplay" {
        n133 = Unbundle By Name(w390) -> ("DerStationIndex"=w395:i32, "Mode"=w394:bool, "AnalogData"=w393:dbl[][], "station index"=w392:i32, "dataNO."=w391:i32, "Position Refnum"=w382:refnum<vi>)
        n134 = call "Direct Control Data Interaction.vi"("mode"=enum16{"Init", "read", "write"}."read") -> ("电流值输出"=w386:sgl[], "玻璃当前Hall输出"=w387:i64[])  [unwired: 8 in, 1 out]
        n135 = Index Array(array=w387, index=w395) -> (element=w381:i64)
        n136 = case shown="假" w394 {
          tunnel: w393 -> [w419 _]
          tunnel: w392 -> [w418 _]
          tunnel: w391 -> [w417 _]
          tunnel: w390 -> [w416 w425]
          tunnel: [w413 w425] -> w389
          tunnel: w382 -> [w403 _]
          tunnel: w381 -> [w402 _]
          frame False {
            n137 = property class="Ctl"(reference=w403) -> (reference out=w411:refnum<vi>, "Value"=w410:variant)  [unwired: 1 in, 1 out]
            n138 = call "EOL All-Station AI Circular Data Buffer.vi"("station idx"=w418, "Mode"=enum16{"Initialize", "Read", "Write"}."Read") -> ("Data Read (Samp-Ro, Ch-Col)"=w423:sgl[][])  [unwired: 9 in]
            n139 = Array Size(array=w423) -> (size(s)=w422:i32[])
            n140 = Variant To Data(type=cluster{string, i32}[] [], Variant=w410) -> (data=w409:cluster{string, i32}[])  [unwired: 1 in, 1 out]
            n141 = Index Array(array=w422) -> (element=w424:i32)  [unwired: 1 in]
            n142 = Index Array(array=w409, index=1 ("索引")) -> (element=w412:cluster{string, i32})
            n143 = Add(x=w424, y=w417) -> (x+y=w414:i32)
            n144 = Bundle("Position", "玻璃当前Hall"=w402) -> (w407:cluster{string, "玻璃当前Hall":i64})  [unwired: 1 in]
            n145 = Replace Array Subset(array=w419, new element=w423, index (row)=w417, index (col)=0 ("disabled index (col)")) -> (w415:dbl[][])
            n146 = Build Array(w407, w412) -> (w408:cluster{string, "玻璃当前Hall":i64}[])
            n147 = Bundle By Name(cluster=w416, "AnalogData"=w415, "dataNO."=w414) -> (w413:T7)
            n148 = property class="Ctl"(reference=w411, "Value"=w408) -> ()  [unwired: 1 in, 2 out]
          }
          frame True {
          }
        }
        n149 = Index Array(array=w386, index=w395) -> (element=w385:sgl)
        n150 = case shown="真" "Display" {
          tunnel: w381 -> [_ w401]
          tunnel: w385 -> [_ w400]
          frame False {
          }
          frame True {
            n151 = Bundle("玻璃当前Hall"=w401, "玻璃当前Hall"=w400) -> (→"波形图表":cluster{"玻璃当前Hall":i64, "玻璃当前Hall":sgl})  [unwired: 1 in]
            "霍尔位置" <- w401
          }
        }
        n152 = call <vilib>:"Add State(s) to Queue__JKI_lib_State_Machine.vi"("State(s) in (\"\")"=w396) -> ("States Out"=w397:string)  [unwired: 14 in]
      }
      frame "---------- Macro ----------" {
        # "Do not put any code in this frame.\n(It is a separator no-op. You can make a copy of this frame to create a new Macro frame)"
        n153 = call <vilib>:"Add State(s) to Queue__JKI_lib_State_Machine.vi"("State(s) in (\"\")"=w430) -> ("States Out"=w429:string)  [unwired: 14 in]
      }
      frame "Macro: Initialize" {
        w433 = "Data: Initialize\nData: Initialize 2\nInitialize Core Data\nUI: Initialize\nUI: Front Panel State >> Open"  # Data: Initialize Data: Initialize 2 Initialize Core Data UI: Initialize UI: Front Panel State >> Open
        # "Initialization Macro\n(This is called once, when the VI starts)"
        n154 = call <vilib>:"Add State(s) to Queue__JKI_lib_State_Machine.vi"("State(s) in Front (\"\")"=w433, "State(s) in (\"\")"=w436) -> ("States Out"=w435:string)  [unwired: 13 in]
      }
      frame "Macro: Exit" {
        # "Exit Macro\n(This is called once, when the VI exits)"
        n155 = Unbundle By Name(w446) -> ("Core.Close Panel on Exit?"=w445:bool)
        n156 = Format Into String(format string="Data: Cleanup>>%s\nExit", w438) -> (resulting string=w437:string)  [unwired: 2 in, 1 out]
        n157 = Select(t="UI: Front Panel State >> Close", s=w445, f="") -> (s? t:f=w442:string)
        n158 = call <vilib>:"Add State(s) to Queue__JKI_lib_State_Machine.vi"("State(s) in (\"\")"=w442, "State(s) at Back (\"\")"=w437) -> ("States Out"=w441:string)  [unwired: 13 in]
        n159 = call <vilib>:"Add State(s) to Queue__JKI_lib_State_Machine.vi"("State(s) in Front (\"\")"=w441, "State(s) in (\"\")"=w449) -> ("States Out"=w448:string)  [unwired: 13 in]
      }
      frame "---------- Manual CMD ----------" {
        # "Template Separator\n(You can make a copy of, or modify, this frame)"
        n160 = call <vilib>:"Add State(s) to Queue__JKI_lib_State_Machine.vi"("State(s) in (\"\")"=w454) -> ("States Out"=w453:string)  [unwired: 14 in]
      }
      frame "ManualCMD-DirectControl FullOpen" {
        w455 = 16 ("禁用的索引 (列)")
        # "Your code here.\n(You can make a copy of, or modify, this frame)"
        n161 = Unbundle By Name(w458) -> ("DerStationIndex"=w462:i32)
        n162 = call "Direct Motor Remote Param.vi"("mode"=Direct_Value_Mode."write Msend cmd", "M-send cmd in"=w455, "index"=w462) -> ()  [unwired: 16 in, 9 out]
        n163 = Tick Count (ms)() -> (millisecond timer value=w457:u32)
        n164 = Bundle By Name(cluster=w458, "RunTime"=w457) -> (w456:T7)
        n165 = Format Into String(format string="ManualCMD-WaitMotorStop>>0x%02x", w455) -> (resulting string=w459:string)  [unwired: 2 in, 1 out]
        n166 = call <vilib>:"Add State(s) to Queue__JKI_lib_State_Machine.vi"("State(s) in (\"\")"=w466, "State(s) at Back (\"\")"=w459) -> ("States Out"=w465:string)  [unwired: 13 in]
      }
      frame "ManualCMD-DirectControl FullClose" {
        w467 = 32 ("禁用的索引 (列)")
        # "Your code here.\n(You can make a copy of, or modify, this frame)"
        n167 = Unbundle By Name(w470) -> ("DerStationIndex"=w474:i32)
        n168 = call "Direct Motor Remote Param.vi"("mode"=Direct_Value_Mode."write Msend cmd", "M-send cmd in"=w467, "index"=w474) -> ()  [unwired: 16 in, 9 out]
        n169 = Tick Count (ms)() -> (millisecond timer value=w468:u32)
        n170 = Bundle By Name(cluster=w470, "RunTime"=w468) -> (w469:T7)
        n171 = Format Into String(format string="ManualCMD-WaitMotorStop>>0x%02x", w467) -> (resulting string=w471:string)  [unwired: 2 in, 1 out]
        n172 = call <vilib>:"Add State(s) to Queue__JKI_lib_State_Machine.vi"("State(s) in (\"\")"=w478, "State(s) at Back (\"\")"=w471) -> ("States Out"=w477:string)  [unwired: 13 in]
      }
      frame "ManualCMD-DirectControl ManualFullOpen" {
        # "Your code here.\n(You can make a copy of, or modify, this frame)"
        n173 = Unbundle By Name(w488) -> ("DerStationIndex"=w490:i32, "Mode"=w482:bool, "Action Switch"=w481:T1, "Stop Switch"=w480:T1)
        n174 = call "Direct Motor Remote Param.vi"("mode"=Direct_Value_Mode."write Msend cmd", "M-send cmd in"=48 ("禁用的索引 (列)"), "index"=w490) -> ()  [unwired: 16 in, 9 out]
        n175 = case shown="假" w482 {
          tunnel: w485 -> [_ w500]
          tunnel: [w496 w499] -> w484
          tunnel: w481 -> [w498 _]
          tunnel: w480 -> [w497 _]
          tunnel: w479 -> [w495 _]
          frame False {
            # "auto"
            n176 = call "ManualModeNextState.vi"("current state"=w495, "Stop2 Switch"=w497, "Stop1 Switch"=w498) -> ("next state"=w496:string)  [unwired: 8 in]
          }
          frame True {
            # "debug"
            n177 = Concatenate Strings(">>", w500) -> (w499:string)
          }
        }
        n178 = Tick Count (ms)() -> (millisecond timer value=w487:u32)
        n179 = Bundle By Name(cluster=w488, "RunTime"=w487) -> (w486:T7)
        n180 = call <vilib>:"Add State(s) to Queue__JKI_lib_State_Machine.vi"("State(s) in (\"\")"=w494, "State(s) at Back (\"\")"=w484) -> ("States Out"=w493:string)  [unwired: 13 in]
      }
      frame "ManualCMD-DirectControl ManualFullClose" {
        # "Your code here.\n(You can make a copy of, or modify, this frame)"
        n181 = Unbundle By Name(w511) -> ("DerStationIndex"=w513:i32, "Mode"=w506:bool, "Stop Switch"=w505:T1, "Action Switch"=w504:T1)
        n182 = call "Direct Motor Remote Param.vi"("mode"=Direct_Value_Mode."write Msend cmd", "M-send cmd in"=64 ("禁用的索引 (列)"), "index"=w513) -> ()  [unwired: 16 in, 9 out]
        n183 = case shown="假" w506 {
          tunnel: w507 -> [_ w523]
          tunnel: [w519 w522] -> w503
          tunnel: w505 -> [w521 _]
          tunnel: w504 -> [w520 _]
          tunnel: w502 -> [w518 _]
          frame False {
            # "auto"
            n184 = call "ManualModeNextState.vi"("current state"=w518, "Stop2 Switch"=w520, "Stop1 Switch"=w521) -> ("next state"=w519:string)  [unwired: 8 in]
          }
          frame True {
            # "debug"
            n185 = Concatenate Strings(">>", w523) -> (w522:string)
          }
        }
        n186 = Tick Count (ms)() -> (millisecond timer value=w510:u32)
        n187 = Bundle By Name(cluster=w511, "RunTime"=w510) -> (w509:T7)
        n188 = call <vilib>:"Add State(s) to Queue__JKI_lib_State_Machine.vi"("State(s) in (\"\")"=w517, "State(s) at Back (\"\")"=w503) -> ("States Out"=w516:string)  [unwired: 13 in]
      }
      frame "ManualCMD-DirectControl Teach" {
        w525 = 80 ("禁用的索引 (列)")
        # "Your code here.\n(You can make a copy of, or modify, this frame)"
        n189 = Unbundle By Name(w528) -> ("DerStationIndex"=w532:i32)
        n190 = call "Direct Motor Remote Param.vi"("mode"=Direct_Value_Mode."write Msend cmd", "M-send cmd in"=w525, "index"=w532) -> ()  [unwired: 16 in, 9 out]
        n191 = Tick Count (ms)() -> (millisecond timer value=w527:u32)
        n192 = Bundle By Name(cluster=w528, "RunTime"=w527) -> (w526:T7)
        n193 = Format Into String(format string="ManualCMD-WaitMotorStop>>0x%02x", w525) -> (resulting string=w529:string)  [unwired: 2 in, 1 out]
        n194 = call <vilib>:"Add State(s) to Queue__JKI_lib_State_Machine.vi"("State(s) in (\"\")"=w536, "State(s) at Back (\"\")"=w529) -> ("States Out"=w535:string)  [unwired: 13 in]
      }
      frame "ManualCMD-DirectControl SetParam" {
        # "Your code here.\n(You can make a copy of, or modify, this frame)"
        n195 = Unbundle By Name(w544) -> ("DerStationIndex"=w541:i32, "Hall Positions"=w539:i32[])
        n196 = call "Direct Motor Remote Param.vi"("position in"=w539, "mode"=Direct_Value_Mode."write position", "index"=w541) -> ()  [unwired: 16 in, 9 out]
        n197 = Tick Count (ms)() -> (millisecond timer value=w543:u32)
        n198 = Wait (ms)(milliseconds to wait=u32 50 ("等待时间（毫秒）")) -> ()  [unwired: 1 out]
        n199 = Bundle By Name(cluster=w544, "RunTime"=w543) -> (w542:T7)
        n200 = call <vilib>:"Add State(s) to Queue__JKI_lib_State_Machine.vi"("State(s) in Front (\"\")"="ManualCMD-Check Param", "State(s) in (\"\")"=w548) -> ("States Out"=w547:string)  [unwired: 13 in]
      }
      frame "ManualCMD-Check Param" {
        # "Your code here.\n(You can make a copy of, or modify, this frame)"
        n201 = Unbundle By Name(w560) -> ("DerStationIndex"=w557:i32, "Hall Positions"=w555:i32[])
        n202 = call "Direct Motor Remote Param.vi"("mode"=Direct_Value_Mode."read", "index"=w557) -> ("position out"=w554:i64[])  [unwired: 17 in, 8 out]
        n203 = Equal?(x=w555, y=w554) -> (x = y?=w553:bool[])
        n204 = And Array Elements(Boolean array=w553) -> (logical AND=w549:bool)
        n205 = Select(t="", s=w549, f="ManualCMD-DirectControl SetParam") -> (s? t:f=w550:string)
        n206 = Tick Count (ms)() -> (millisecond timer value=w559:u32)
        n207 = local write "结果"(w549) -> ()
        n208 = Bundle By Name(cluster=w560, "RunTime"=w559, "test state"=w549) -> (w558:T7)
        n209 = call <vilib>:"Add State(s) to Queue__JKI_lib_State_Machine.vi"("State(s) in Front (\"\")"=w550, "State(s) in (\"\")"=w564) -> ("States Out"=w563:string)  [unwired: 13 in]
      }
      frame "ManualCMD-WaitMotorStop" {
        w567 = FALSE ("值")
        # "Your code here.\n(You can make a copy of, or modify, this frame)"
        n210 = Unbundle By Name(w585) -> ("Mode"=w572:bool, "Exit Refnum"=w586:refnum<vi>, "RunTime"=w587:i32, "DerStationIndex"=w589:i32, "Action Switch"=w566:T1, "Stop Switch"=w565:T1)
        n211 = call "Direct Motor Remote Param.vi"("mode"=Direct_Value_Mode."read", "index"=w589) -> ("recevie cmd out"=w568:u32, "ErrorString out"=w582:string)  [unwired: 17 in, 7 out]
        n212 = case shown="\"0x10\"" w570 {
          tunnel: w568 -> [_ w597 w609 w621 w633]
          tunnel: w587 -> [_ w605 w617 w629 w641]
          tunnel: [TRUE w600 w612 w624 w636] -> w575
          tunnel: [FALSE w599 w611 w623 w635] -> w573
          tunnel: ["program exception - %s" "Motor Stoped in Sunshade FullOpen：%s" "Motor Stoped in Sunshade FullClose：%s" "Motor Stoped in Sunshade Teach：%s" "Motor Stoped in Sunshade GotoPosition：%s"] -> w581
          frame Default {
          }
          frame "0x10" {
            n213 = Tick Count (ms)() -> (millisecond timer value=w606:u32)
            n214 = Subtract(x=w606, y=w605) -> (x-y=w604:u32)
            n215 = Equal?(x=17, y=w597) -> (x = y?=w602:bool)
            n216 = Equal?(x=18, y=w597) -> (x = y?=w599:bool)
            n217 = Greater?(x=w604, y=u32 3000) -> (0:w601:bool)
            n218 = And(x=w601, y=w602) -> (x .and. y?=w600:bool)
          }
          frame "0x20" {
            n219 = Tick Count (ms)() -> (millisecond timer value=w618:u32)
            n220 = Subtract(x=w618, y=w617) -> (x-y=w616:u32)
            n221 = Equal?(x=33, y=w609) -> (x = y?=w614:bool)
            n222 = Equal?(x=34, y=w609) -> (x = y?=w611:bool)
            n223 = Greater?(x=w616, y=u32 3000) -> (0:w613:bool)
            n224 = And(x=w613, y=w614) -> (x .and. y?=w612:bool)
          }
          frame "0x50" {
            n225 = Tick Count (ms)() -> (millisecond timer value=w630:u32)
            n226 = Subtract(x=w630, y=w629) -> (x-y=w628:u32)
            n227 = Equal?(x=81, y=w621) -> (x = y?=w626:bool)
            n228 = Equal?(x=82, y=w621) -> (x = y?=w623:bool)
            n229 = Greater?(x=w628, y=u32 3000) -> (0:w625:bool)
            n230 = And(x=w625, y=w626) -> (x .and. y?=w624:bool)
          }
          frame "0x60" {
            n231 = Tick Count (ms)() -> (millisecond timer value=w642:u32)
            n232 = Subtract(x=w642, y=w641) -> (x-y=w640:u32)
            n233 = Equal?(x=97, y=w633) -> (x = y?=w638:bool)
            n234 = Equal?(x=98, y=w633) -> (x = y?=w635:bool)
            n235 = Greater?(x=w640, y=u32 3000) -> (0:w637:bool)
            n236 = And(x=w637, y=w638) -> (x .and. y?=w636:bool)
          }
        }
        n237 = property class="Bool (严格)" props=["Value"](reference=w586) -> ()  [unwired: 1 in, 3 out]
        n238 = Compound Arithmetic op=OR ("复合运算")(w567, w575, w573) -> (w571:bool)
        n239 = Format Into String(format string=w581, w582) -> (resulting string=w580:string)  [unwired: 2 in, 1 out]
        n240 = Or(x=w575, y=w567) -> (x .or. y?=w576:bool)
        n241 = Select(t=w580, s=w575, f="Test Abord") -> (s? t:f=w578:string)
        n242 = Bundle By Name(cluster=w579, "source"=w578, "status"=w576, "code"=212) -> (w577:errorcluster)
        n243 = call "GetNextSatae.vi"("Stop2 Switch"=w565, "Stop1 Switch"=w566, "输入字符串"=w570, "Done"=w571, "debug"=w572) -> ("after"=w569:string)  [unwired: 6 in]
        n244 = Bundle By Name(cluster=w585, "test state"=w573) -> (w584:T7)
        n245 = local write "结果"(w573) -> ()
        n246 = call <vilib>:"Add State(s) to Queue__JKI_lib_State_Machine.vi"("State(s) in (\"\")"=w592, "State(s) at Back (\"\")"=w569) -> ("States Out"=w591:string)  [unwired: 13 in]
      }
      frame "ManualCMD-SwitchRemoteStop" {
        n247 = Unbundle By Name(w656) -> ("DerStationIndex"=w644:i32)
        n248 = call "Direct Motor Remote Param.vi"("remote Stop in"=TRUE, "mode"=Direct_Value_Mode."write RS", "index"=w644) -> ()  [unwired: 16 in, 9 out]
        n249 = Bundle By Name(cluster=w655, "status"=TRUE, "source"="Test Abord at manual operator action", "code"=212) -> (w654:errorcluster)
        n250 = call <vilib>:"Add State(s) to Queue__JKI_lib_State_Machine.vi"("State(s) in (\"\")"=w653, "State(s) at Back (\"\")"="Macro: Exit") -> ("States Out"=w652:string)  [unwired: 13 in]
      }
      frame "ManualCMD-MotorStop" {
        n251 = flat-sequence {
          tunnel: w659 -> [w665]
          frame #0 {
            n252 = Unbundle By Name(w665) -> ("DerStationIndex"=w664:i32)
            n253 = call "Direct Motor Remote Param.vi"("send cmd in"=u32 0 ("cmd in"), "mode"=Direct_Value_Mode."write Msend cmd", "index"=w664) -> ()  [unwired: 16 in, 9 out]
          }
          frame #1 {
            n254 = Wait (ms)(milliseconds to wait=u32 300 ("等待时间（毫秒）")) -> ()  [unwired: 1 out]
          }
        }
        n255 = call <vilib>:"Add State(s) to Queue__JKI_lib_State_Machine.vi"("State(s) in (\"\")"=w658) -> ("States Out"=w661:string)  [unwired: 14 in]
      }
      frame "---------- Auto CMD ----------" {
        # "Template Separator\n(You can make a copy of, or modify, this frame)"
        n256 = call <vilib>:"Add State(s) to Queue__JKI_lib_State_Machine.vi"("State(s) in (\"\")"=w671) -> ("States Out"=w670:string)  [unwired: 14 in]
      }
      frame "CMD-DirectControl Teach" {
        w675 = 80 ("禁用的索引 (列)")
        # "Your code here.\n(You can make a copy of, or modify, this frame)"
        n257 = Unbundle By Name(w674) -> ("DerStationIndex"=w679:i32)
        n258 = call "Direct Motor Remote Param.vi"("send cmd in"=w675, "mode"=Direct_Value_Mode."write send cmd", "index"=w679) -> ()  [unwired: 16 in, 9 out]
        n259 = Tick Count (ms)() -> (millisecond timer value=w673:u32)
        n260 = Bundle By Name(cluster=w674, "RunTime"=w673) -> (w672:T7)
        n261 = Format Into String(format string="CMD-WaitMotorStop>>0x%02x", w675) -> (resulting string=w676:string)  [unwired: 2 in, 1 out]
        n262 = call <vilib>:"Add State(s) to Queue__JKI_lib_State_Machine.vi"("State(s) in (\"\")"=w683, "State(s) at Back (\"\")"=w676) -> ("States Out"=w682:string)  [unwired: 13 in]
      }
      frame "CMD-DirectControl FullOpen" {
        w688 = 16 ("禁用的索引 (列)")
        # "Your code here.\n(You can make a copy of, or modify, this frame)"
        n263 = Unbundle By Name(w686) -> ("DerStationIndex"=w691:i32)
        n264 = call "Direct Motor Remote Param.vi"("send cmd in"=w688, "mode"=Direct_Value_Mode."write send cmd", "index"=w691) -> ()  [unwired: 16 in, 9 out]
        n265 = Tick Count (ms)() -> (millisecond timer value=w685:u32)
        n266 = Bundle By Name(cluster=w686, "RunTime"=w685) -> (w684:T7)
        n267 = Format Into String(format string="CMD-WaitMotorStop>>0x%02x", w688) -> (resulting string=w687:string)  [unwired: 2 in, 1 out]
        n268 = call <vilib>:"Add State(s) to Queue__JKI_lib_State_Machine.vi"("State(s) in (\"\")"=w695, "State(s) at Back (\"\")"=w687) -> ("States Out"=w694:string)  [unwired: 13 in]
      }
      frame "CMD-DirectControl FullClose" {
        w699 = 32 ("禁用的索引 (列)")
        # "Your code here.\n(You can make a copy of, or modify, this frame)"
        n269 = Unbundle By Name(w698) -> ("DerStationIndex"=w703:i32)
        n270 = call "Direct Motor Remote Param.vi"("send cmd in"=w699, "mode"=Direct_Value_Mode."write send cmd", "index"=w703) -> ()  [unwired: 16 in, 9 out]
        n271 = Tick Count (ms)() -> (millisecond timer value=w696:u32)
        n272 = Bundle By Name(cluster=w698, "RunTime"=w696) -> (w697:T7)
        n273 = Format Into String(format string="CMD-WaitMotorStop>>0x%02x", w699) -> (resulting string=w700:string)  [unwired: 2 in, 1 out]
        n274 = call <vilib>:"Add State(s) to Queue__JKI_lib_State_Machine.vi"("State(s) in (\"\")"=w707, "State(s) at Back (\"\")"=w700) -> ("States Out"=w706:string)  [unwired: 13 in]
      }
      frame "CMD-DirectControl Goto Position" {
        w711 = 96 ("禁用的索引 (列)")
        # "Your code here.\n(You can make a copy of, or modify, this frame)"
        n275 = Unbundle By Name(w710) -> ("DerStationIndex"=w715:i32)
        n276 = call "Direct Motor Remote Param.vi"("send cmd in"=w711, "mode"=Direct_Value_Mode."write send cmd", "index"=w715) -> ()  [unwired: 16 in, 9 out]
        n277 = Tick Count (ms)() -> (millisecond timer value=w709:u32)
        n278 = Bundle By Name(cluster=w710, "RunTime"=w709) -> (w708:T7)
        n279 = Format Into String(format string="CMD-WaitMotorStop>>0x%02x", w711) -> (resulting string=w712:string)  [unwired: 2 in, 1 out]
        n280 = call <vilib>:"Add State(s) to Queue__JKI_lib_State_Machine.vi"("State(s) in (\"\")"=w719, "State(s) at Back (\"\")"=w712) -> ("States Out"=w718:string)  [unwired: 13 in]
      }
      frame "CMD-DirectControl SetParam" {
        # "Your code here.\n(You can make a copy of, or modify, this frame)"
        n281 = Unbundle By Name(w727) -> ("DerStationIndex"=w724:i32, "Hall Positions"=w722:i32[])
        n282 = call "Direct Motor Remote Param.vi"("position in"=w722, "mode"=Direct_Value_Mode."write position", "index"=w724) -> ()  [unwired: 16 in, 9 out]
        n283 = Tick Count (ms)() -> (millisecond timer value=w726:u32)
        n284 = Wait (ms)(milliseconds to wait=u32 50 ("等待时间（毫秒）")) -> ()  [unwired: 1 out]
        n285 = Bundle By Name(cluster=w727, "RunTime"=w726) -> (w725:T7)
        n286 = call <vilib>:"Add State(s) to Queue__JKI_lib_State_Machine.vi"("State(s) in Front (\"\")"="CMD-Check Param", "State(s) in (\"\")"=w731) -> ("States Out"=w730:string)  [unwired: 13 in]
      }
      frame "CMD-Check Param" {
        # "Your code here.\n(You can make a copy of, or modify, this frame)"
        n287 = Unbundle By Name(w743) -> ("DerStationIndex"=w740:i32, "Hall Positions"=w738:i32[])
        n288 = call "Direct Motor Remote Param.vi"("mode"=Direct_Value_Mode."read", "index"=w740) -> ("position out"=w737:i64[])  [unwired: 17 in, 8 out]
        n289 = Equal?(x=w738, y=w737) -> (x = y?=w736:bool[])
        n290 = And Array Elements(Boolean array=w736) -> (logical AND=w732:bool)
        n291 = Select(t="", s=w732, f="CMD-DirectControl SetParam") -> (s? t:f=w733:string)
        n292 = Tick Count (ms)() -> (millisecond timer value=w742:u32)
        n293 = local write "结果"(w732) -> ()
        n294 = Bundle By Name(cluster=w743, "RunTime"=w742, "test state"=w732) -> (w741:T7)
        n295 = call <vilib>:"Add State(s) to Queue__JKI_lib_State_Machine.vi"("State(s) in Front (\"\")"=w733, "State(s) in (\"\")"=w747) -> ("States Out"=w746:string)  [unwired: 13 in]
      }
      frame "CMD-WaitMotorStop" {
        # "Your code here.\n(You can make a copy of, or modify, this frame)"
        n296 = Unbundle By Name(w769) -> ("Exit Refnum"=w770:refnum<vi>, "RunTime"=w771:i32, "DerStationIndex"=w773:i32)  [unwired: 2 out]
        n297 = call "Direct Motor Remote Param.vi"("mode"=Direct_Value_Mode."read", "index"=w773) -> ("recevie cmd out"=w755:u32, "ErrorString out"=w766:string)  [unwired: 17 in, 7 out]
        n298 = case shown="\"0x50\"" w749 {
          tunnel: w755 -> [_ w781 w793 w805 w817]
          tunnel: w771 -> [_ w789 w801 w813 w825]
          tunnel: [TRUE w784 w796 w808 w820] -> w759
          tunnel: [FALSE w783 w795 w807 w819] -> w756
          tunnel: ["program exception - %s" "Motor Stoped in Sunshade FullOpen：%s" "Motor Stoped in Sunshade FullClose：%s" "Motor Stoped in Sunshade Teach：%s" "Motor Stoped in Sunshade GotoPosition：%s"] -> w765
          frame Default {
          }
          frame "0x10" {
            n299 = Tick Count (ms)() -> (millisecond timer value=w790:u32)
            n300 = Subtract(x=w790, y=w789) -> (x-y=w788:u32)
            n301 = Equal?(x=17, y=w781) -> (x = y?=w786:bool)
            n302 = Equal?(x=18, y=w781) -> (x = y?=w783:bool)
            n303 = Greater?(x=w788, y=u32 3000) -> (0:w785:bool)
            n304 = And(x=w785, y=w786) -> (x .and. y?=w784:bool)
          }
          frame "0x20" {
            n305 = Tick Count (ms)() -> (millisecond timer value=w802:u32)
            n306 = Subtract(x=w802, y=w801) -> (x-y=w800:u32)
            n307 = Equal?(x=33, y=w793) -> (x = y?=w798:bool)
            n308 = Equal?(x=34, y=w793) -> (x = y?=w795:bool)
            n309 = Greater?(x=w800, y=u32 3000) -> (0:w797:bool)
            n310 = And(x=w797, y=w798) -> (x .and. y?=w796:bool)
          }
          frame "0x50" {
            n311 = Tick Count (ms)() -> (millisecond timer value=w814:u32)
            n312 = Subtract(x=w814, y=w813) -> (x-y=w812:u32)
            n313 = Equal?(x=81, y=w805) -> (x = y?=w810:bool)
            n314 = Equal?(x=82, y=w805) -> (x = y?=w807:bool)
            n315 = Greater?(x=w812, y=u32 3000) -> (0:w809:bool)
            n316 = And(x=w809, y=w810) -> (x .and. y?=w808:bool)
          }
          frame "0x60" {
            n317 = Tick Count (ms)() -> (millisecond timer value=w826:u32)
            n318 = Subtract(x=w826, y=w825) -> (x-y=w824:u32)
            n319 = Equal?(x=97, y=w817) -> (x = y?=w822:bool)
            n320 = Equal?(x=98, y=w817) -> (x = y?=w819:bool)
            n321 = Greater?(x=w824, y=u32 3000) -> (0:w821:bool)
            n322 = And(x=w821, y=w822) -> (x .and. y?=w820:bool)
          }
        }
        n323 = property class="Bool (严格)"(reference=w770) -> ("Value"=w758:bool)  [unwired: 1 in, 2 out]
        n324 = Compound Arithmetic op=OR ("复合运算")(w758, w759, w756) -> (w753:bool)
        n325 = Format Into String(format string=w765, w766) -> (resulting string=w764:string)  [unwired: 2 in, 1 out]
        n326 = Select(t=w764, s=w759, f="Test Abord") -> (s? t:f=w762:string)
        n327 = Or(x=w759, y=w758) -> (x .or. y?=w760:bool)
        n328 = Bundle By Name(cluster=w763, "source"=w762, "status"=w760, "code"=212) -> (w761:errorcluster)
        n329 = Format Into String(format string="UI: UpdataDisplay\nCMD-WaitMotorStop>>%s", w749) -> (resulting string=w752:string)  [unwired: 2 in, 1 out]
        n330 = Format Into String(format string="Macro: Exit>>%s", w749) -> (resulting string=w748:string)  [unwired: 2 in, 1 out]
        n331 = Bundle By Name(cluster=w769, "test state"=w756) -> (w768:T7)
        n332 = local write "结果"(w756) -> ()
        n333 = Select(t=w748, s=w753, f=w752) -> (s? t:f=w751:string)
        n334 = call <vilib>:"Add State(s) to Queue__JKI_lib_State_Machine.vi"("State(s) in (\"\")"=w776, "State(s) at Back (\"\")"=w751) -> ("States Out"=w775:string)  [unwired: 13 in]
      }
    }
  }
  n335 = Unbundle By Name(w5) -> ("Error"=→"Error":string, "test state"=→"结果":bool, "motion string"=→"motion str":string, "AnalogData"=→"AnalogData out":dbl[][])
